vi "ke37xx List to Array.vi"(4 "List":string, 7 "Separator (,)":string=",") -> (0 "Output Number Array":dbl[](array[numeric]) format="%.2f", 3 "Output String Array":string[](array[string]))   [LabVIEW 2009, in "Keithley 3700 Series.lvlib"]
doc: "Given a List of strings separated by a Separator, this VI returns the List as a String Array. If the strings are numbers, a Number Array is also returned."
uses:
  <instrlib>/Keithley 3706/Keithley 3700 Series.lvlib
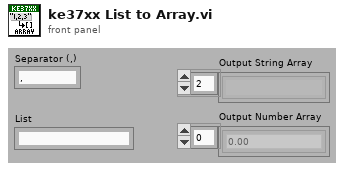
[diagram p1: front panel]
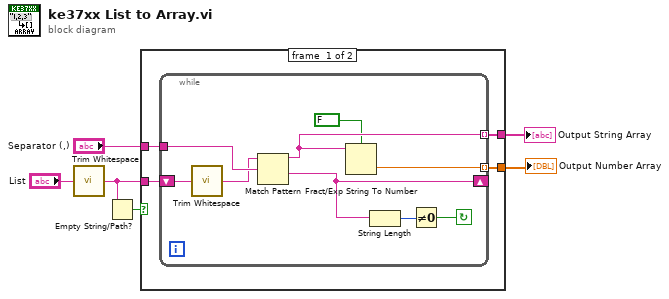
[diagram p0: block diagram]
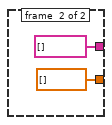
[diagram p2: hidden frame]
diagram:
  n1 = call <vilib>:"Trim Whitespace.vi"("string"="List") -> ("trimmed string"=w2:string)  [unwired: 1 in]
  n2 = Empty String/Path?(string/path=w2) -> (empty?=w1:bool)
  n3 = case shown="False" w1 {
    tunnel: "Separator (,)" -> [w10 _]
    tunnel: [w9 string[] []] -> w5
    tunnel: [w8 dbl[] []] -> w4
    tunnel: w2 -> [w7 _]
    frame #0 {
      n4 = while {
        tunnel: w10 -> [w14]
        tunnel: [w15] -> w9 mode=indexing
        tunnel: [w17] -> w8 mode=indexing
        shift-left: w7 -> [w12]
        shift-right: [w16] -> _
        stop <- w19 continue-if-true
        n5 = call <vilib>:"Trim Whitespace.vi"("string"=w12) -> ("trimmed string"=w11:string)  [unwired: 1 in]
        n6 = Match Pattern(string=w11, regular expression=w14) -> (before substring=w15:string, after substring=w16:string)  [unwired: 3 out]
        n7 = Fract/Exp String To Number(use system decimal point (T)=FALSE, string=w15) -> (number=w17:dbl)  [unwired: 3 out]
        n8 = String Length(string=w16) -> (length=w18:i32)
        n9 = Not Equal To 0?(x=w18) -> (x != 0?=w19:bool)
      }
    }
    frame #1 {
    }
  }
  "Output String Array" <- w5
  "Output Number Array" <- w4
